vi "FormProductsTable.vi"() -> ()   [LabVIEW 2013]
uses:
  resultShow.vi
  S7Ref.vi
panel:
  in  "判定设定 2":string[][](table)
  in  "参数设定 2":string[][](table)
  in  "判定设定":string[][](table)
  in  "参数设定":string[][](table)
  in  "功能选择":T1
  in  "产品选择":bool
  in  "产品删除":bool
  in  "产品更新":bool
  in  "产品注册":bool
  in  "产品":string(combo)
  # "磨合速度"
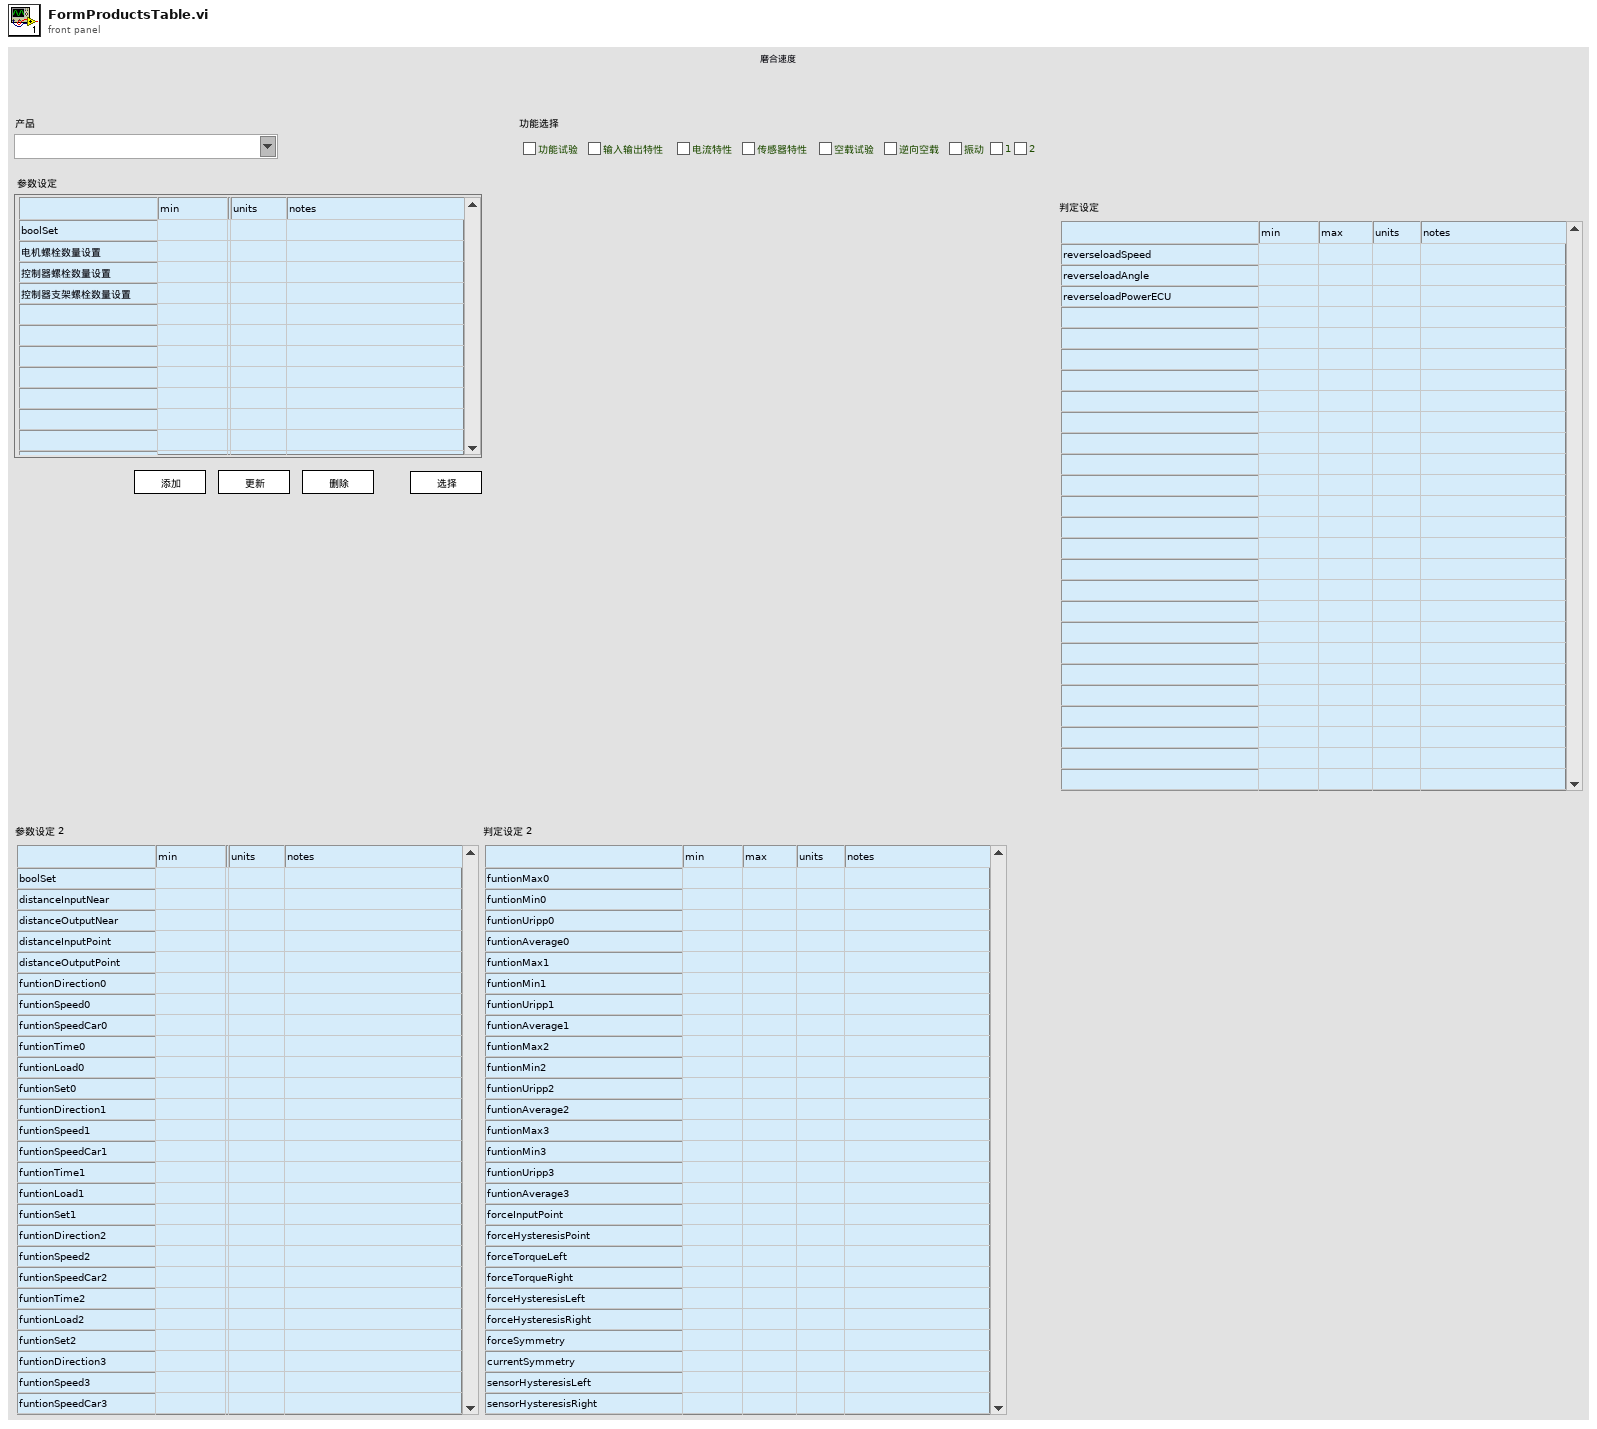
[diagram p1: front panel]
types:
  T1 = cluster{"功能试验":bool, "输入输出特性":bool, "电流特性":bool, "传感器特性":bool, "空载试验":bool, "逆向空载":bool, "振动":bool, "1":bool, "2":bool}
  T2 = enum16{"selectdata", "selectsave", "selectlist", "selectshow"}
  T3 = enum8{"Enabled", "Disabled", "Disabled and Grayed Out"}
  T4 = cluster{"Boolean array[0]":bool, "Boolean array[1]":bool, "Boolean array[2]":bool, "Boolean array[3]":bool, "Boolean array[4]":bool, "Boolean array[5]":bool, "Boolean array[6]":bool, "Boolean array[7]":bool, "Boolean array[8]":bool}
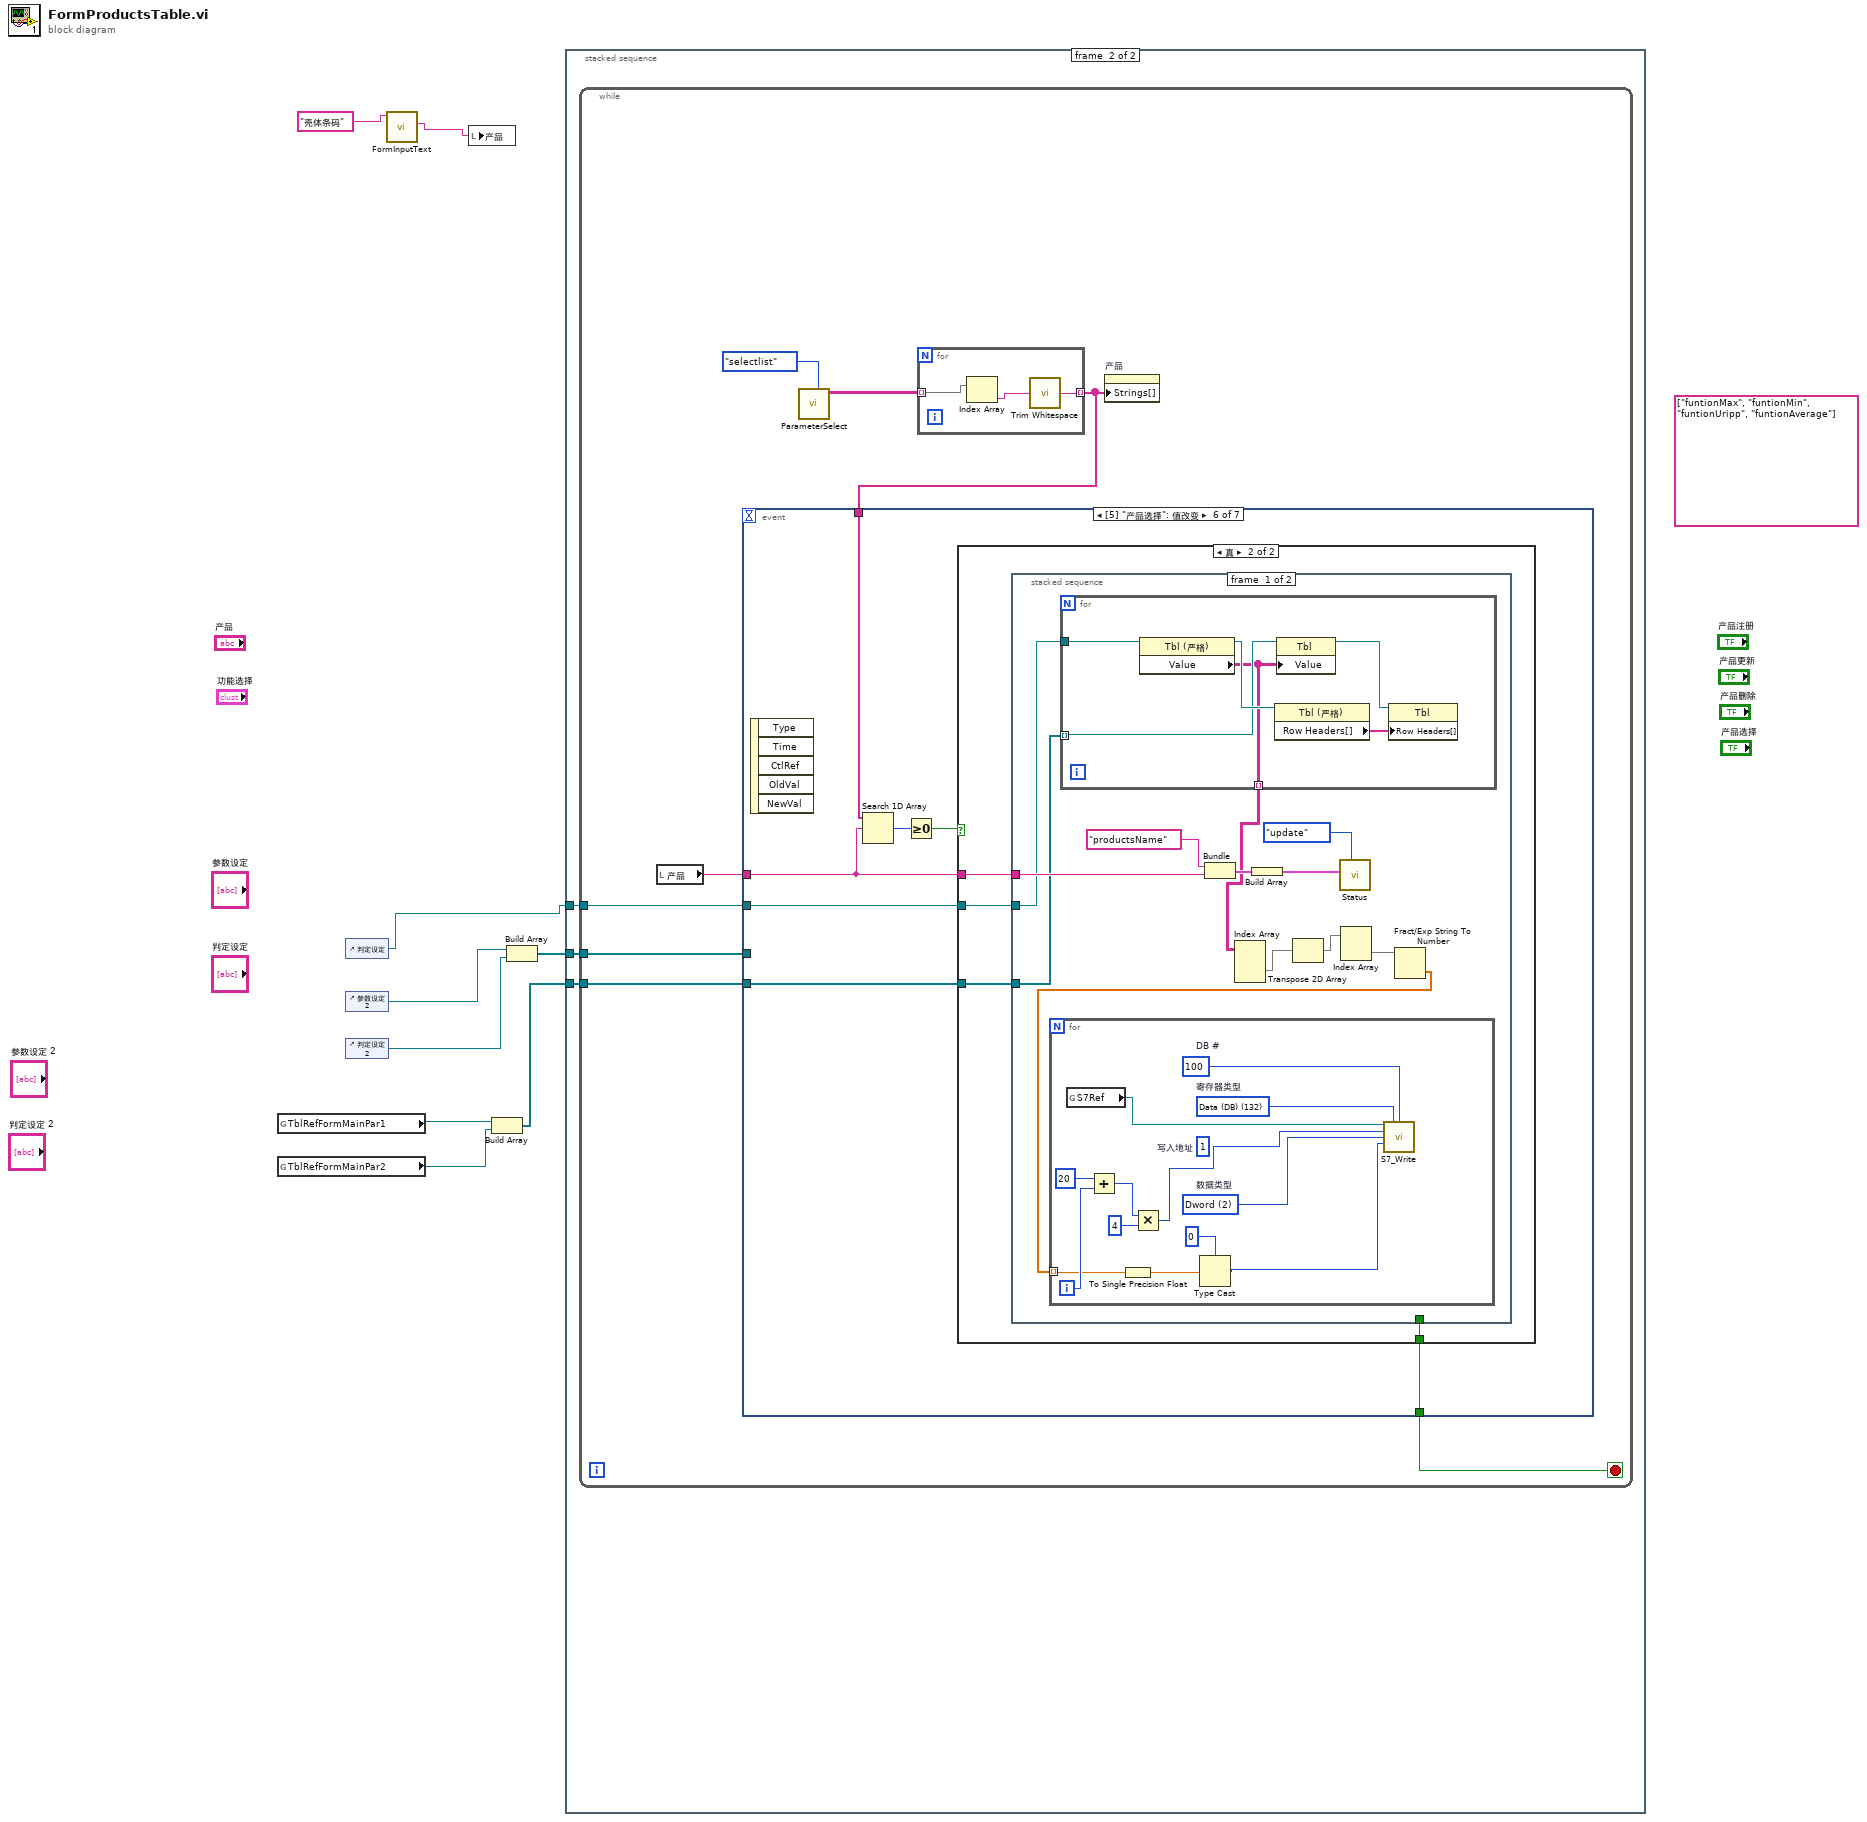
[diagram p0: block diagram]
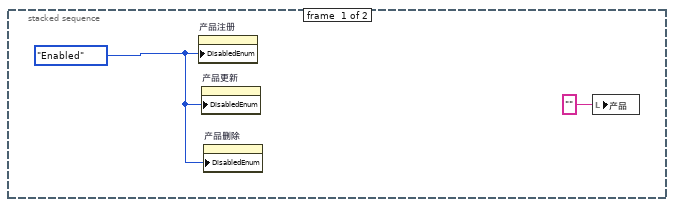
[diagram p2: hidden frame]
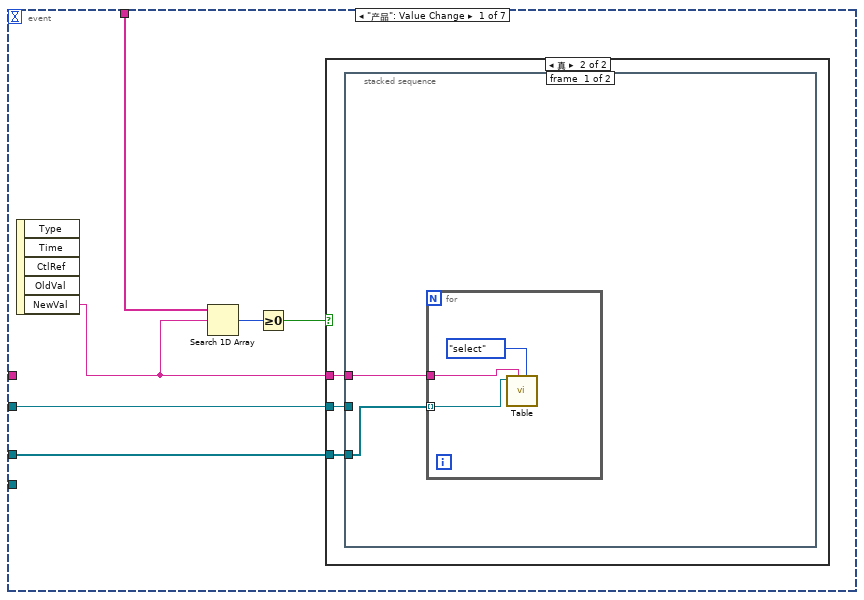
[diagram p3: hidden frame]
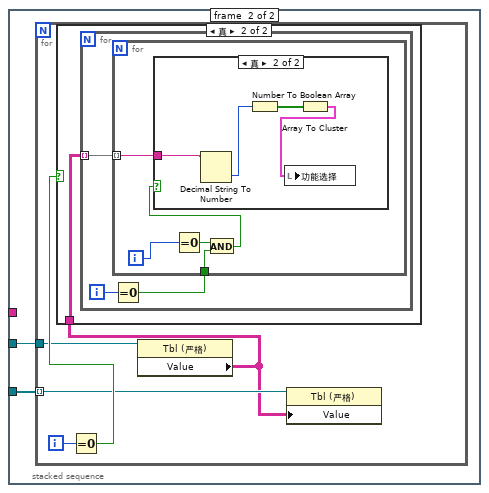
[diagram p5: hidden frame]
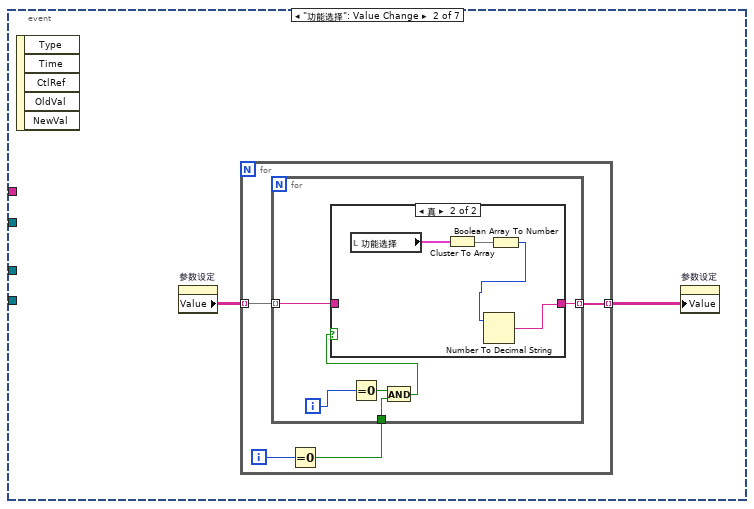
[diagram p8: hidden frame]
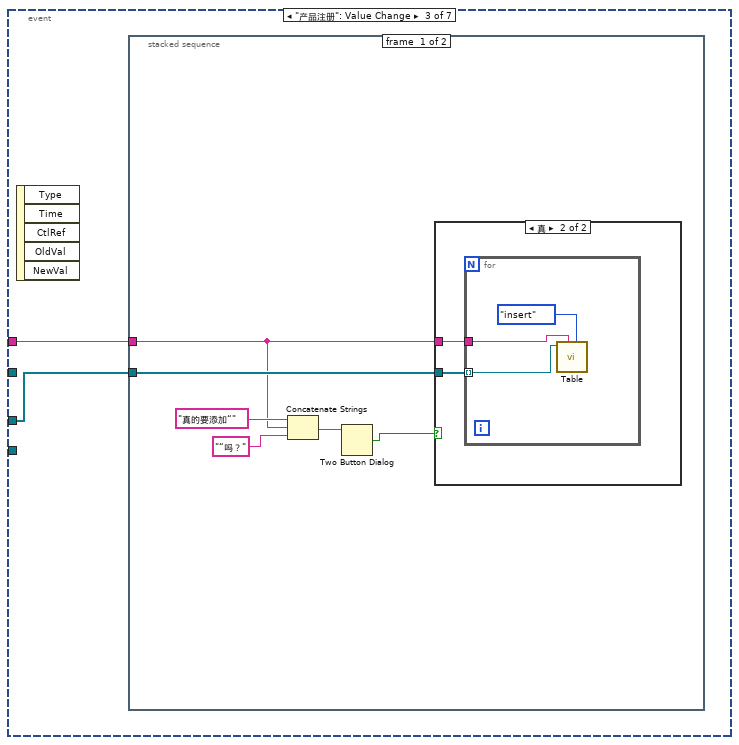
[diagram p10: hidden frame]
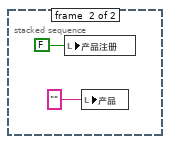
[diagram p12: hidden frame]
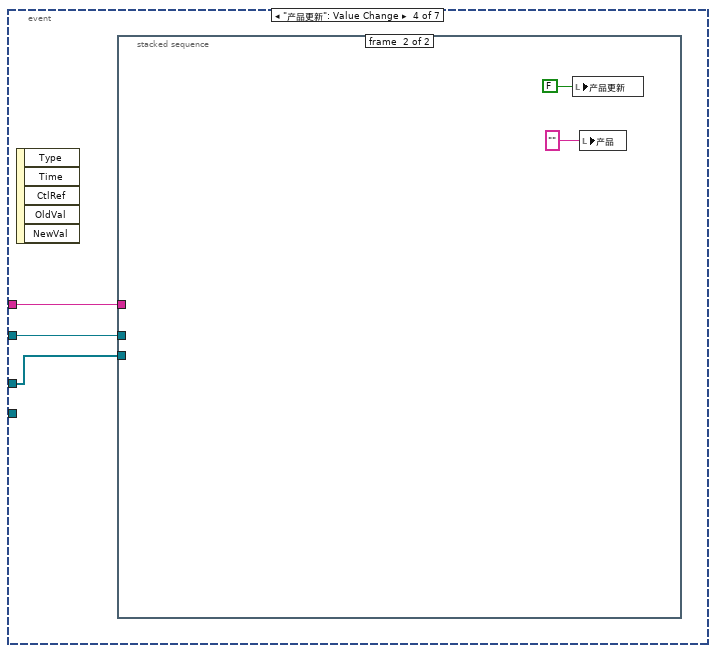
[diagram p13: hidden frame]
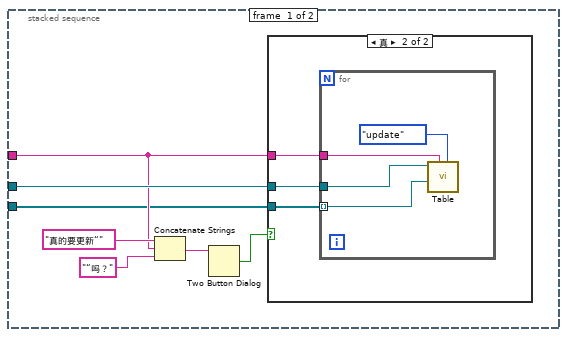
[diagram p14: hidden frame]
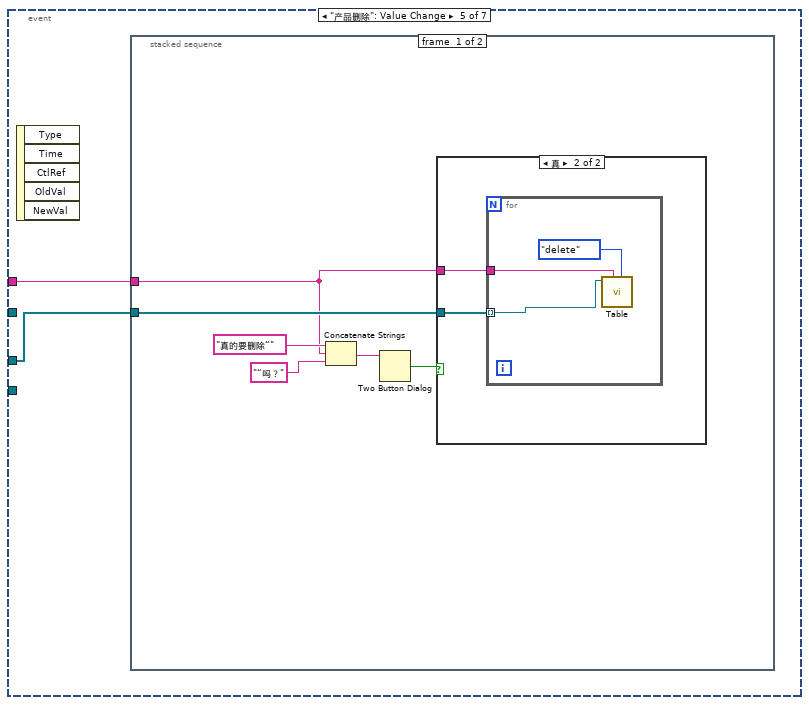
[diagram p16: hidden frame]
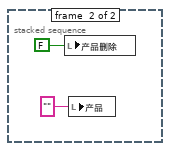
[diagram p18: hidden frame]
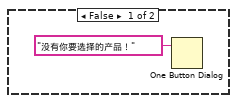
[diagram p19: hidden frame]
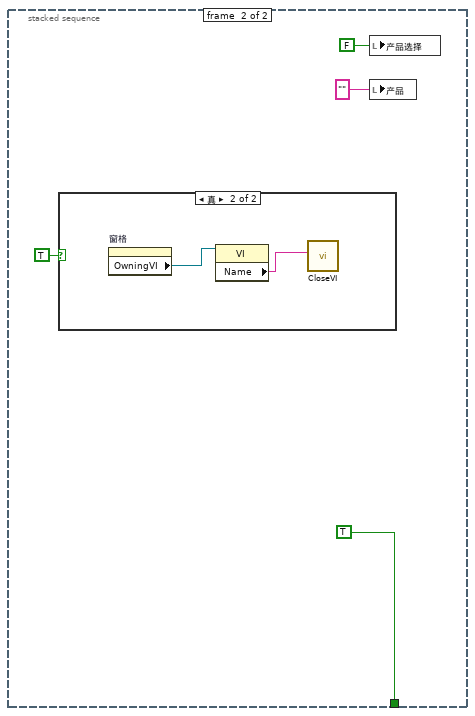
[diagram p20: hidden frame]
diagram:
  (unwired) string[] ["funtionMax", "funtionMin", "funtionUripp", "funtionAverage"] ("字符串[]")
  n1 = global read "resultShow.vi" "TblRefFormMainPar1"() -> (w8:refnum<vi>)
  n2 = global read "resultShow.vi" "TblRefFormMainPar2"() -> (w7:refnum<vi>)
  n3 = control-ref of="判定设定"() -> (w1:refnum<vi>)
  n4 = control-ref of="参数设定 2"() -> (w5:refnum<vi>)
  n5 = control-ref of="判定设定 2"() -> (w6:refnum<vi>)
  n6 = call "FormInputText.vi"("提示信息"="壳体条码") -> ("返回"=w3:string)  [unwired: 10 in]
  n7 = local write "产品"(w3) -> ()
  n8 = Build Array(w8, w7) -> (w9:refnum<vi>[])
  n9 = Build Array(w5, w6) -> (w4:refnum<vi>[])
  n10 = stacked-sequence {
    tunnel: w1 -> [_ w14]
    tunnel: w9 -> [_ w13]
    tunnel: w4 -> [_ w12]
    frame #0 {
      w10 = T3."Enabled" ("禁用")
      n11 = property on="产品注册" class="Bool (严格)"("DisabledEnum"=w10) -> ()  [unwired: 2 in, 2 out]
      n12 = property on="产品更新" class="Bool (严格)"("DisabledEnum"=w10) -> ()  [unwired: 2 in, 2 out]
      n13 = property on="产品删除" class="Bool (严格)"("DisabledEnum"=w10) -> ()  [unwired: 2 in, 2 out]
      n14 = local write "产品"("" ("y")) -> ()
    }
    frame #1 {
      n15 = while {
        tunnel: w14 -> [w19]
        tunnel: w13 -> [w16]
        tunnel: w12 -> [w15]
        stop <- w22 stop-if-true
        n16 = local read "产品"() -> (w21:string)
        n17 = call "ParameterSelect.vi"("模式"=T2."selectlist") -> ("dataOutAll"=w18:string[][])  [unwired: 5 in, 5 out]
        n18 = for {
          tunnel: w18 -> [w24] mode=indexing
          tunnel: [w25] -> w20 mode=indexing
          n19 = Index Array(array=w24) -> (element=w23:string)  [unwired: 1 in]
          n20 = call <vilib>:"Trim Whitespace.vi"("string"=w23) -> ("trimmed string"=w25:string)  [unwired: 1 in]
        }
        n21 = event shown="[5] \"产品选择\": 值改变" {
          selector: _ -> [_ _ _ _ _ _ _]
          dyn-events: _ -> [_ _ _ _ _ _ _]
          timeout: _ -> [_ _ _ _ _ _ _]
          tunnel: [_ _ _ _ _ w132 w175] -> w22
          tunnel: w19 -> [w31 _ _ w94 _ w127 _]
          tunnel: w21 -> [_ _ w78 w93 w112 w130 _]
          tunnel: w20 -> [w30 _ _ _ _ w131 _]
          tunnel: w16 -> [_ _ _ _ _ w126 _]
          tunnel: w15 -> [w26 _ w77 w92 w111 _ _]
          event "产品": Value Change {
            n22 = event-data() -> ("NewVal"=w28:string)  [unwired: 1 in, 4 out]
            n23 = Search 1D Array(1D array=w30, element=w28) -> (index of element=w29:i32)  [unwired: 1 in]
            n24 = Greater Or Equal To 0?(x=w29) -> (x >= 0?=w27:bool)
            n25 = case shown="真" w27 {
              tunnel: w31 -> [_ w34]
              tunnel: w28 -> [_ w33]
              tunnel: w26 -> [_ w32]
              frame False {
              }
              frame True {
                n26 = stacked-sequence {
                  tunnel: w34 -> [_ w41]
                  tunnel: w33 -> [w36 _]
                  tunnel: w32 -> [w35 w40]
                  frame #0 {
                    n27 = for {
                      tunnel: w35 -> [w39] mode=indexing
                      tunnel: w36 -> [w38]
                      n28 = call "Table.vi"("模式"=enum16{"select", "insert", "update", "delete"}."select", "productsName"=w38, "Table"=w39) -> ()  [unwired: 9 in]
                    }
                  }
                  frame #1 {
                    n29 = for {
                      tunnel: w41 -> [w44]
                      tunnel: w40 -> [w43] mode=indexing
                      i -> [w45]
                      n30 = Equal To 0?(x=w45) -> (x = 0?=w46:bool)
                      n31 = property on="属性节点" class="Tbl (严格)"(reference=w44) -> ("Value"=w42:string[][])  [unwired: 1 in, 2 out]
                      n32 = case shown="真" w46 {
                        tunnel: w42 -> [_ w47]
                        frame False {
                        }
                        frame True {
                          n33 = for {
                            tunnel: w47 -> [w48] mode=indexing
                            i -> [w50]
                            n34 = Equal To 0?(x=w50) -> (x = 0?=w49:bool)
                            n35 = for {
                              tunnel: w48 -> [w52] mode=indexing
                              tunnel: w49 -> [w53]
                              i -> [w54]
                              n36 = Equal To 0?(x=w54) -> (x = 0?=w55:bool)
                              n37 = And(x=w55, y=w53) -> (x .and. y?=w51:bool)
                              n38 = case shown="真" w51 {
                                tunnel: w52 -> [_ w57]
                                frame False {
                                }
                                frame True {
                                n39 = Decimal String To Number(string=w57) -> (number=w56:i32)  [unwired: 2 in, 1 out]
                                n40 = Number To Boolean Array(number=w56) -> (Boolean array=w59:bool[])
                                n41 = Array To Cluster(array=w59) -> (cluster=w58:T4)
                                n42 = local write "功能选择"(w58) -> ()
                                }
                              }
                            }
                          }
                        }
                      }
                      n43 = property on="属性节点" class="Tbl (严格)"(reference=w43, "Value"=w42) -> ()  [unwired: 1 in, 2 out]
                    }
                  }
                }
              }
            }
          }
          event "功能选择": Value Change {
            n44 = event-data() -> ()  [unwired: 1 in, 5 out]
            n45 = property on="参数设定" class="Tbl (严格)"() -> ("Value"=w61:string[][])  [unwired: 2 in, 2 out]
            n46 = for {
              tunnel: w61 -> [w65] mode=indexing
              tunnel: [w62] -> w60 mode=indexing
              i -> [w64]
              n47 = Equal To 0?(x=w64) -> (x = 0?=w63:bool)
              n48 = for {
                tunnel: w65 -> [w67] mode=indexing
                tunnel: w63 -> [w69]
                tunnel: [w68] -> w62 mode=indexing
                i -> [w70]
                n49 = Equal To 0?(x=w70) -> (x = 0?=w71:bool)
                n50 = And(x=w71, y=w69) -> (x .and. y?=w66:bool)
                n51 = case shown="真" w66 {
                  tunnel: [w72 w73] -> w68
                  tunnel: w67 -> [w72 _]
                  frame False {
                  }
                  frame True {
                    n52 = local read "功能选择"() -> (w76:T1)
                    n53 = Cluster To Array(cluster=w76) -> (array=w75:bool[])
                    n54 = Boolean Array To Number(Boolean array=w75) -> (number=w74:u32)
                    n55 = Number To Decimal String(number=w74) -> (decimal integer string=w73:string)  [unwired: 1 in]
                  }
                }
              }
            }
            n56 = property on="参数设定" class="Tbl (严格)"("Value"=w60) -> ()  [unwired: 2 in, 2 out]
          }
          event "产品注册": Value Change {
            n57 = event-data() -> ()  [unwired: 1 in, 5 out]
            n58 = stacked-sequence {
              tunnel: w77 -> [w84 _]
              tunnel: w78 -> [w79 _]
              frame #0 {
                n59 = Concatenate Strings("真的要添加“" ("消息"), w79, "“吗？" ("消息")) -> (w81:string)
                n60 = Two Button Dialog(message=w81) -> (T button?=w80:bool)  [unwired: 2 in]
                n61 = case shown="真" w80 {
                  tunnel: w84 -> [_ w86]
                  tunnel: w79 -> [_ w85]
                  frame False {
                  }
                  frame True {
                    n62 = for {
                      tunnel: w86 -> [w88] mode=indexing
                      tunnel: w85 -> [w87]
                      n63 = call "Table.vi"("模式"=enum16{"select", "insert", "update", "delete"}."insert", "productsName"=w87, "Table"=w88) -> ()  [unwired: 9 in]
                    }
                  }
                }
              }
              frame #1 {
                n64 = local write "产品注册"(FALSE ("产品注册")) -> ()
                n65 = local write "产品"("") -> ()
              }
            }
          }
          event "产品更新": Value Change {
            n66 = event-data() -> ()  [unwired: 1 in, 5 out]
            n67 = stacked-sequence {
              tunnel: w94 -> [w101 _]
              tunnel: w93 -> [w96 _]
              tunnel: w92 -> [w95 _]
              frame #0 {
                n68 = Concatenate Strings("真的要更新“" ("消息"), w96, "“吗？" ("消息")) -> (w98:string)
                n69 = Two Button Dialog(message=w98) -> (T button?=w97:bool)  [unwired: 2 in]
                n70 = case shown="真" w97 {
                  tunnel: w101 -> [_ w104]
                  tunnel: w96 -> [_ w103]
                  tunnel: w95 -> [_ w102]
                  frame False {
                  }
                  frame True {
                    n71 = for {
                      tunnel: w104 -> [w107]
                      tunnel: w103 -> [w106]
                      tunnel: w102 -> [w105] mode=indexing
                      n72 = call "Table.vi"("模式"=enum16{"select", "insert", "update", "delete"}."update", "productsName"=w106, "Table 2"=w105, "Table"=w107) -> ()  [unwired: 8 in]
                    }
                  }
                }
              }
              frame #1 {
                n73 = local write "产品更新"(FALSE ("产品注册")) -> ()
                n74 = local write "产品"("") -> ()
              }
            }
          }
          event "产品删除": Value Change {
            n75 = event-data() -> ()  [unwired: 1 in, 5 out]
            n76 = stacked-sequence {
              tunnel: w111 -> [w118 _]
              tunnel: w112 -> [w113 _]
              frame #0 {
                n77 = Concatenate Strings("真的要删除“" ("消息"), w113, "“吗？" ("消息")) -> (w115:string)
                n78 = Two Button Dialog(message=w115) -> (T button?=w114:bool)  [unwired: 2 in]
                n79 = case shown="真" w114 {
                  tunnel: w118 -> [_ w120]
                  tunnel: w113 -> [_ w119]
                  frame False {
                  }
                  frame True {
                    n80 = for {
                      tunnel: w120 -> [w122] mode=indexing
                      tunnel: w119 -> [w121]
                      n81 = call "Table.vi"("模式"=enum16{"select", "insert", "update", "delete"}."delete", "productsName"=w121, "Table"=w122) -> ()  [unwired: 9 in]
                    }
                  }
                }
              }
              frame #1 {
                n82 = local write "产品删除"(FALSE ("产品删除")) -> ()
                n83 = local write "产品"("" ("products_name_in")) -> ()
              }
            }
          }
          event "产品选择": Value Change {
            n84 = event-data() -> ()  [unwired: 1 in, 5 out]
            n85 = Search 1D Array(1D array=w131, element=w130) -> (index of element=w129:i32)  [unwired: 1 in]
            n86 = Greater Or Equal To 0?(x=w129) -> (x >= 0?=w128:bool)
            n87 = case shown="真" w128 {
              tunnel: [_ w137] -> w132
              tunnel: w130 -> [_ w136]
              tunnel: w127 -> [_ w135]
              tunnel: w126 -> [_ w134]
              frame False {
                n88 = One Button Dialog(message="没有你要选择的产品！" ("消息")) -> ()  [unwired: 1 in, 1 out]
              }
              frame True {
                n89 = stacked-sequence {
                  tunnel: w136 -> [w147 _]
                  tunnel: [_ TRUE ("产品删除")] -> w137
                  tunnel: w135 -> [w140 _]
                  tunnel: w134 -> [w141 _]
                  frame #0 {
                    n90 = for {
                      tunnel: w141 -> [w151] mode=indexing
                      tunnel: w140 -> [w152]
                      tunnel: [w150] -> w139 mode=indexing
                      n91 = property on="属性节点" class="Tbl (严格)"(reference=w152) -> (reference out=w154:refnum<vi>, "Value"=w150:string[][])  [unwired: 1 in, 1 out]
                      n92 = property on="属性节点" class="Tbl (严格)"(reference=w154) -> ("Row Headers[]"=w153:string[])  [unwired: 1 in, 2 out]
                      n93 = property on="属性节点" class="Tbl"(reference=w151, "Value"=w150) -> (reference out=w155:refnum<vi>)  [unwired: 1 in, 1 out]
                      n94 = property on="属性节点" class="Tbl"(reference=w155, "Row Headers[]"=w153) -> ()  [unwired: 1 in, 2 out]
                    }
                    n95 = Bundle("name"="productsName", "产品"=w147) -> (w146:cluster{"name":string, "产品":string})  [unwired: 1 in]
                    n96 = Index Array(array=w139) -> (element=w138:string[][])  [unwired: 3 in]
                    n97 = Build Array(w146) -> (w145:cluster{"name":string, "产品":string}[])
                    n98 = Transpose 2D Array(2D array=w138) -> (transposed array=w142:string[][])
                    n99 = call "Status.vi"("模式"=enum16{"select", "insert", "update", "delete"}."update", "nameData"=w145) -> ()  [unwired: 9 in, 1 out]
                    n100 = Index Array(array=w142) -> (element=w144:string[])  [unwired: 2 in]
                    n101 = Fract/Exp String To Number(string=w144) -> (number=w143:dbl[])  [unwired: 3 in, 1 out]
                    n102 = for {
                      tunnel: w143 -> [w156] mode=indexing
                      i -> [w160]
                      w167 = u16 2 items=["byte", "word", "Dword"]  # 数据类型
                      (unwired) u32 1  # 写入地址
                      w166 = u16 100  # DB #
                      w168 = u8 132 items=["I/O (P)"=128, "Input (I)"=129, "Output (Q)"=130, "Bit Memory (M)"=131, "Data (DB)"=132, "Instance Data (DI)"=133, "Local Data (L)"=134, "Predecessor Local Data (VL)"=135]  # 寄存器类型
                      n103 = global read "S7Ref.vi" "S7Ref"() -> (w162:refnum<k5>)
                      n104 = Add(x=20 ("y"), y=w160) -> (x+y=w159:i32)
                      n105 = To Single Precision Float(number=w156) -> (single precision float=w157:sgl)
                      n106 = Multiply(x=w159, y=4) -> (x*y=w164:i32)
                      n107 = Type Cast(type=u32 0, x=w157) -> (*(type *) &x=w163:u32)
                      n108 = call "S7_Write.vi"("TCP"=w162, "寄存器类型"=w168, "DB #"=w166, "写入地址"=w164, "数据类型"=w167, "写入数据"=w163) -> ()  [unwired: 7 in, 3 out]
                    }
                  }
                  frame #1 {
                    n109 = case shown="真" TRUE {
                      frame False {
                      }
                      frame True {
                        n110 = property on="窗格" class="Pane"() -> ("OwningVI"=w174:refnum<vi>)  [unwired: 2 in, 2 out]
                        n111 = property on="属性节点" class="VI"(reference=w174) -> ("Name"=w173:string)  [unwired: 1 in, 2 out]
                        n112 = call "CloseVI.vi"("名称或相对路径"=w173) -> ()  [unwired: 10 in, 1 out]
                      }
                    }
                    n113 = local write "产品选择"(FALSE ("产品删除")) -> ()
                    n114 = local write "产品"("") -> ()
                  }
                }
              }
            }
          }
          event Panel Close? {
            w175 = TRUE
            n115 = event-data() -> ()  [unwired: 1 in, 3 out]
            n116 = Not(x=w175) -> (.not. x?=w176:bool)
            n117 = event-data("Discard?"=w176) -> ()  [unwired: 1 in, 1 out]
          }
        }
        n118 = property on="产品" class="CmbBox"("Strings[]"=w20) -> ()  [unwired: 2 in, 2 out]
      }
    }
  }
